vi "Get COM Ports.vi"(4 "Scan Period":dbl format="%.2f", 5 "Previous Scan Value":dbl format="%.2f", 6 "Present scan array":dbl[](array[numeric]) format="%.2f", 7 "Value to Output":dbl format="%.2f", 8 "Ch Description":T1={"Ch Name"="", "Type"="", "Function"=enum."Analogue Input", "Ch State"=enum."On", "Calibration type"="", "A"=0.0, "B"=0.0, "C"=0.0, "D"=0.0, "Comments"="", "Address"={"Main"=0, "Ch."=0, "Sub"=0, "Port Name"=""}, "String"="", "Duty"=65535} {"Duty" format="%016b"; "D" format="%#_5g"; "C" format="%#_5g"; "B" format="%#_5g"; "A" format="%#_5g"}, 9 "Ch names":string[](array[string])) -> (0 "Scan comment":string, 1 "Output":dbl format="%.3f", 3 "HelpText":string="Add helpful help text here!")   [LabVIEW 2022 SP3]
uses:
  ADAM Client/Sub VIs/ADAM Controls/Ch_description_ADAM.ctl
  ADAM Client/Sub VIs/ADAM Controls/Module_type_ADAM.ctl
  ADAM Client/Sub VIs/ADAM Controls/Function_ADAM.ctl
  ADAM Client/Sub VIs/ADAM Controls/Channel_State.ctl
  ADAM Client/Sub VIs/ADAM Controls/Calib_type_ADAM.ctl
  ADAM Client/Sub VIs/ADAM Controls/Address.ctl
  <vilib>/Instr/_visa.llb/VISA Find Search Mode.ctl
panel:
  out "Aliases only":string[](array[string])
  out "Canonical Names":string[](array[string])
  out "time string":string
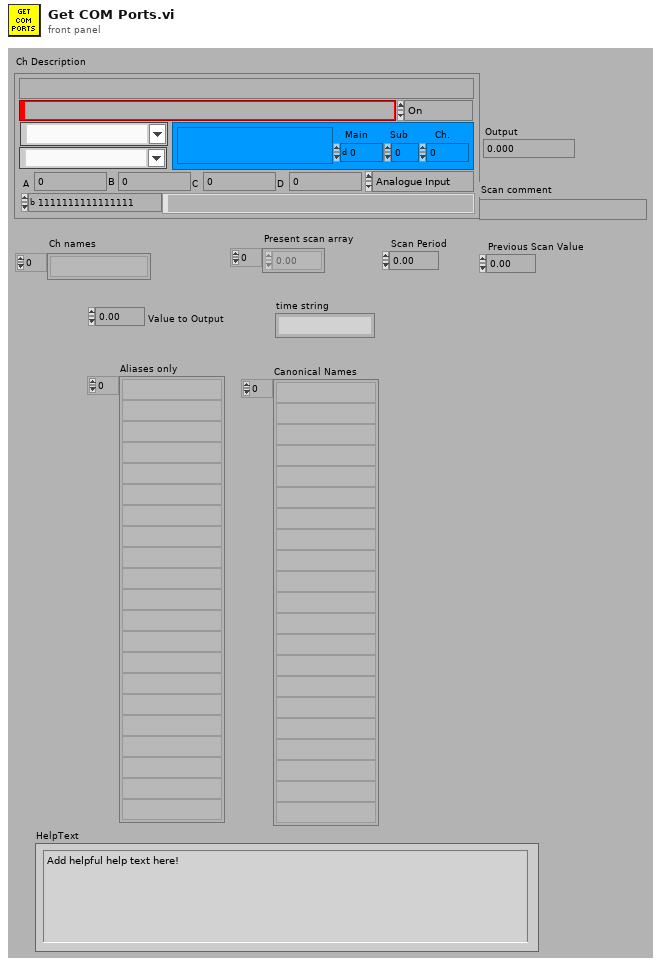
[diagram p1: front panel]
types:
  T1 = typedef "Ch_description_ADAM.ctl" = cluster{"Ch Name":string, "Type":T2, "Function":T3, "Ch State":T4, "Calibration type":T5, "A":dbl, "B":dbl, "C":dbl, "D":dbl, "Comments":string, "Address":T6, "String":string, "Duty":u16}
  T2 = typedef "Module_type_ADAM.ctl" = string
  T3 = typedef "Function_ADAM.ctl" = enum16{"Analogue Input", "Digital Input", "Event counter", "Event rate", "Analogue Output", "Digital Output", "Relay Output"}
  T4 = typedef "Channel_State.ctl" = enum16{"On", "Off", "Always On", "Always Off"}
  T5 = typedef "Calib_type_ADAM.ctl" = string
  T6 = typedef "Address.ctl" = cluster{"Main":i32, "Ch.":i32, "Sub":i32, "Port Name":string}
  T7 = typedef "VISA Find Search Mode.ctl" = u32
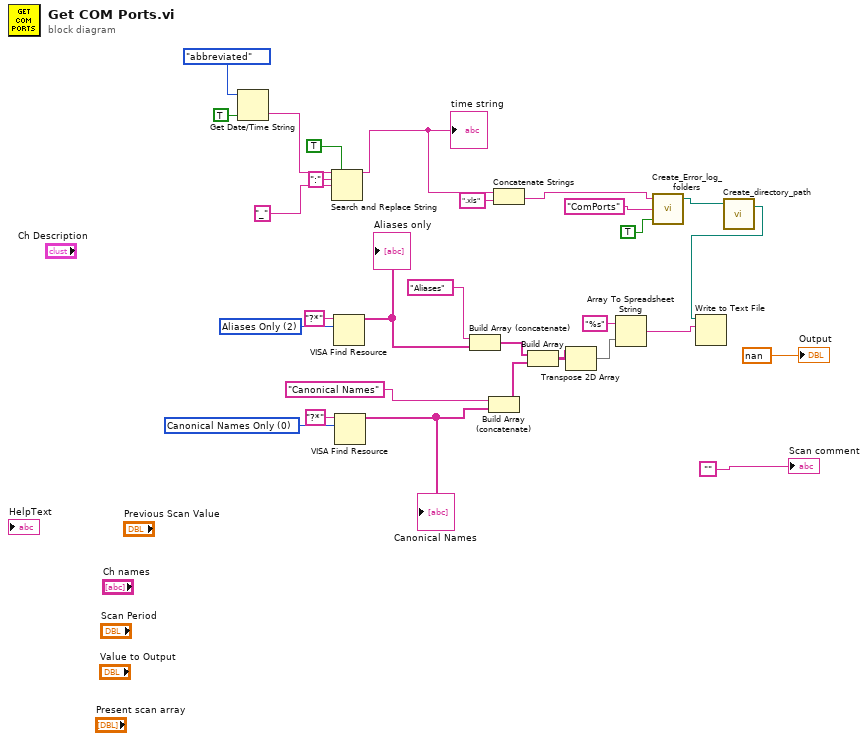
[diagram p0: block diagram]
diagram:
  w19 = T7 0 items=["Canonical Names Only"=0, "Aliases Only"=2, "Include Matching Aliases"=3, "Include All Aliases"=4] ("Search Mode")
  w20 = T7 2 items=["Canonical Names Only"=0, "Aliases Only"=2, "Include Matching Aliases"=3, "Include All Aliases"=4] ("Search Mode")
  n1 = Get Date/Time String(date format (0)=enum16{"short", "long", "abbreviated"}."abbreviated", want seconds? (F)=TRUE) -> (time string=w17:string)  [unwired: 2 out]
  n2 = Search and Replace String(replace all?=TRUE ("replace all? (F)"), input string=w17, search string=":", replace string="_") -> (result string=w13:string)  [unwired: 4 in, 3 out]
  "time string" <- w13
  n3 = VISA Find Resource(10:w20, 11:"?*" ("expression (\"?*\")")) -> (3:w22:string[])  [unwired: 1 in, 2 out]
  "Aliases only" <- w22
  n4 = VISA Find Resource(10:w19, 11:"?*" ("expression (\"?*\")")) -> (3:w6:string[])  [unwired: 1 in, 2 out]
  "Canonical Names" <- w6
  n5 = Build Array (concatenate)("Aliases", w22) -> (w3:string[])
  n6 = Build Array (concatenate)("Canonical Names", w6) -> (w4:string[])
  n7 = Concatenate Strings(w13, ".xls" ("string")) -> (w11:string)
  n8 = Build Array(w3, w4) -> (w2:string[][])
  n9 = Transpose 2D Array(2D array=w2) -> (transposed array=w1:string[][])
  n10 = Array To Spreadsheet String(array=w1, 3:"%s" ("format string")) -> (spreadsheet string=w10:string)  [unwired: 1 in]
  n11 = call "Create_Error_log_folders.vi"("Log Filename"=w11, "Log Folder"="ComPorts", "Per Day Log File?"=TRUE) -> ("Local Log File"=w8:path)  [unwired: 3 in, 1 out]
  n12 = call "Create_directory_path.vi"("Path name"=w8) -> ("Path name Out"=w7:path)  [unwired: 2 in, 1 out]
  n13 = Write to Text File(file (use dialog)=w7, text=w10) -> ()  [unwired: 2 in, 3 out]
  "Output" <- nan
  "Scan comment" <- ""
